vi "Read isOpen.vi"(8 "error in (no error)":errorcluster, 11 "GenericDevice in":refnum<class "GenericDevice.lvclass">) -> (0 "error out":errorcluster, 2 "isOpen":bool, 3 "GenericDevice out":refnum<class "GenericDevice.lvclass">)   [LabVIEW 2023, in "GenericDevice.lvclass"]
uses:
  GenericDevice.lvclass
  GenericDevice.lvclass/GenericDevice.ctl
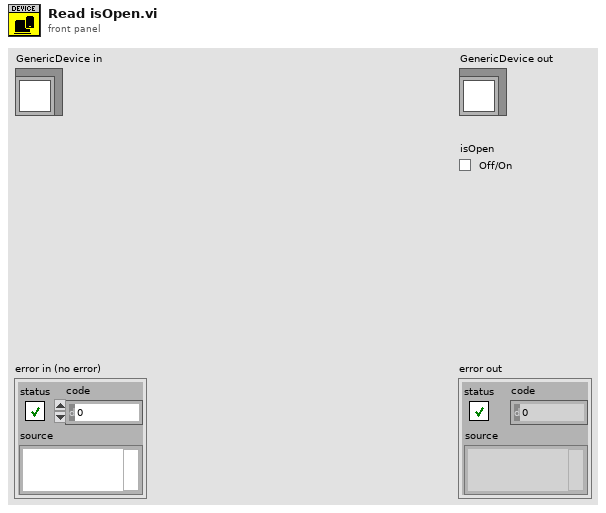
[diagram p1: front panel]
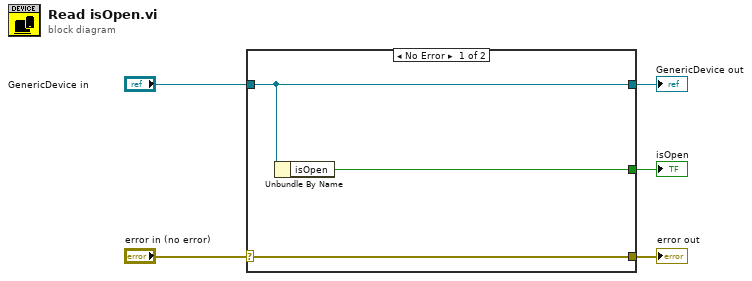
[diagram p0: block diagram]
diagram:
  n1 = case shown="No Error" "error in (no error)" {
    selector: "error in (no error)" -> [w8 w9]
    tunnel: [w8 w9] -> w4
    tunnel: [w7 w10] -> w2
    tunnel: "GenericDevice in" -> [w7 w10]
    tunnel: [w6 _] -> w1
    frame No Error {
      n2 = Unbundle By Name(w7) -> ("isOpen"=w6:bool)
    }
    frame Error {
    }
  }
  "error out" <- w4
  "GenericDevice out" <- w2
  "isOpen" <- w1
